vi "Sort Music Library Display.vi"(7 "Options":T1, 8 "Error In":errorcluster, 10 "Reverse?":bool, 11 "Songs":T2[](array[typedef]) {"Duration (s)" format="%<%M:%S>T"}) -> (0 "Error Out":errorcluster, 3 "Sorted Songs":T2[](array[typedef]) {"Duration (s)" format="%<%M:%S>T"})   [LabVIEW 2015]
uses:
  app/controls/Music Library Element Display.ctl
  MusicElement/Song/Song Duration.ctl
  Music Library Sort Option.ctl
  MusicElement/Song/Song.lvclass
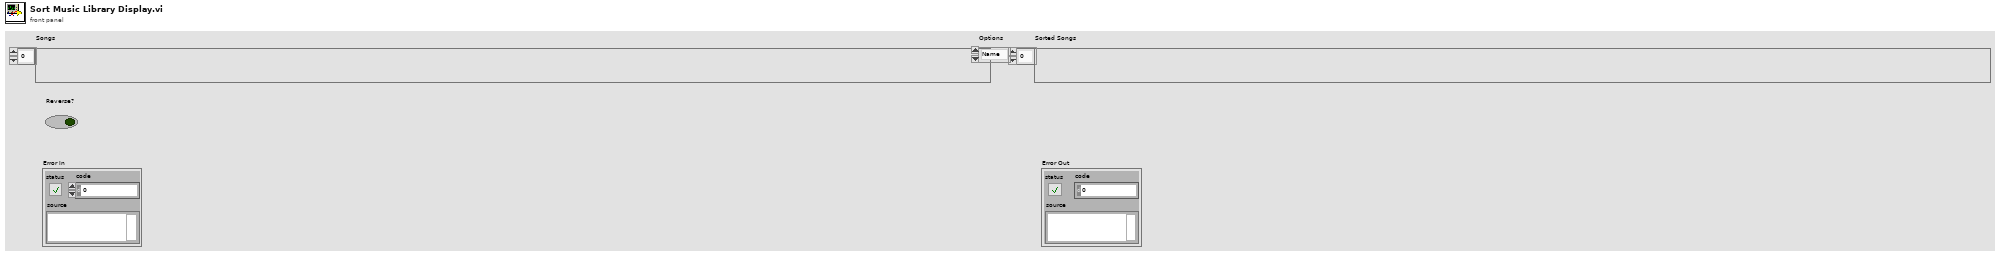
[diagram p1: front panel]
types:
  T1 = typedef "Music Library Sort Option.ctl" = enum16{"Name", "Details", "Time"}
  T2 = typedef "Music Library Element Display.ctl" = cluster{"Name":string, "Details":string, "Duration (s)":T3, "Click":bool}
  T3 = typedef "Song.lvclass/Song Duration.ctl" = timestamp
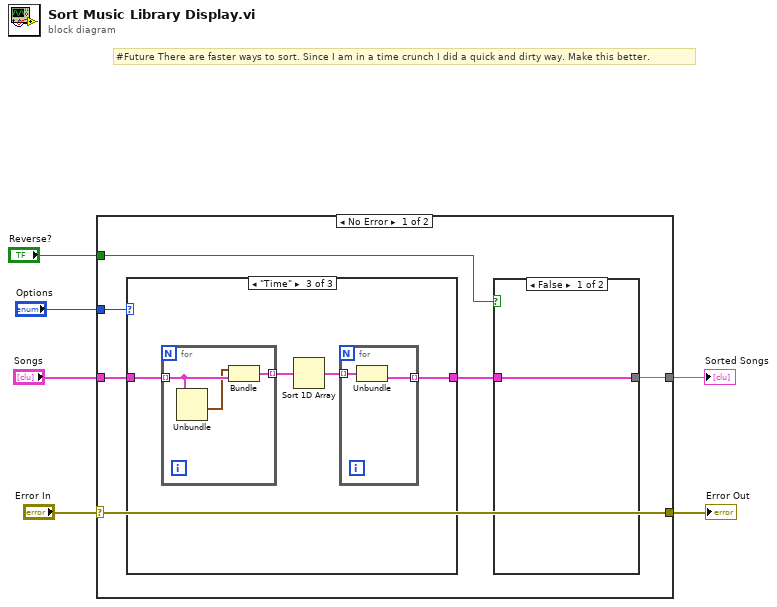
[diagram p0: block diagram]
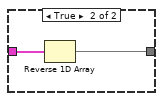
[diagram p2: hidden frame]
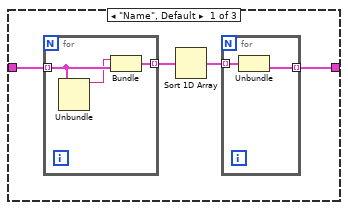
[diagram p3: hidden frame]
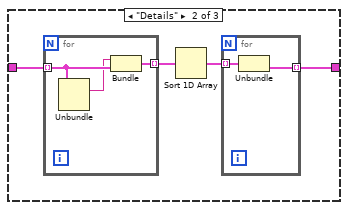
[diagram p4: hidden frame]
diagram:
  # "#Future There are faster ways to sort. Since I am in a time crunch I did a quick and dirty way. Make this better."
  n1 = case shown="No Error" "Error In" {
    selector: "Error In" -> [w9 w44]
    tunnel: [w9 w44] -> w5
    tunnel: "Songs" -> [w12 w43]
    tunnel: "Reverse?" -> [w11 _]
    tunnel: [w8 w43] -> w3
    tunnel: "Options" -> [w7 _]
    frame No Error {
      n2 = case shown="\"Time\"" w7 {
        tunnel: w12 -> [w19 w28 w37]
        tunnel: [w16 w25 w34] -> w10
        frame "Name", Default {
          n3 = for {
            tunnel: w19 -> [w24] mode=indexing
            tunnel: [w23] -> w18 mode=indexing
            n4 = Unbundle(w24) -> ("Name"=w22:string)  [unwired: 3 out]
            n5 = Bundle("Name"=w22, "Element"=w24) -> (w23:cluster{"Name":string, "Element":T2})  [unwired: 1 in]
          }
          n6 = Sort 1D Array(array=w18) -> (sorted array=w17:cluster{"Name":string, "Element":T2}[])
          n7 = for {
            tunnel: w17 -> [w21] mode=indexing
            tunnel: [w20] -> w16 mode=indexing
            n8 = Unbundle(w21) -> ("Element"=w20:T2)  [unwired: 1 out]
          }
        }
        frame "Details" {
          n9 = for {
            tunnel: w28 -> [w33] mode=indexing
            tunnel: [w32] -> w27 mode=indexing
            n10 = Unbundle(w33) -> ("Details"=w31:string)  [unwired: 3 out]
            n11 = Bundle("Details"=w31, "Element"=w33) -> (w32:cluster{"Details":string, "Element":T2})  [unwired: 1 in]
          }
          n12 = Sort 1D Array(array=w27) -> (sorted array=w26:cluster{"Details":string, "Element":T2}[])
          n13 = for {
            tunnel: w26 -> [w30] mode=indexing
            tunnel: [w29] -> w25 mode=indexing
            n14 = Unbundle(w30) -> ("Element"=w29:T2)  [unwired: 1 out]
          }
        }
        frame "Time" {
          n15 = for {
            tunnel: w37 -> [w42] mode=indexing
            tunnel: [w41] -> w36 mode=indexing
            n16 = Unbundle(w42) -> ("Duration (s)"=w40:T3)  [unwired: 3 out]
            n17 = Bundle("Duration (s)"=w40, "Element"=w42) -> (w41:cluster{"Duration (s)":T3, "Element":T2})  [unwired: 1 in]
          }
          n18 = Sort 1D Array(array=w36) -> (sorted array=w35:cluster{"Duration (s)":T3, "Element":T2}[])
          n19 = for {
            tunnel: w35 -> [w39] mode=indexing
            tunnel: [w38] -> w34 mode=indexing
            n20 = Unbundle(w39) -> ("Element"=w38:T2)  [unwired: 1 out]
          }
        }
      }
      n21 = case shown="False" w11 {
        tunnel: w10 -> [w13 w15]
        tunnel: [w13 w14] -> w8
        frame False {
        }
        frame True {
          n22 = Reverse 1D Array(array=w15) -> (reversed array=w14:T2[])
        }
      }
    }
    frame Error {
    }
  }
  "Error Out" <- w5
  "Sorted Songs" <- w3
